vi "Move reports.vi"(11 "source path":path) -> ()   [LabVIEW 2023]
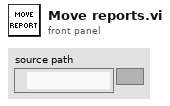
[diagram p1: front panel]
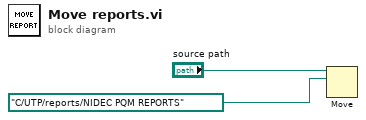
[diagram p0: block diagram]
diagram:
  n1 = Move(source path="source path", 10:path "C:/UTP/reports/NIDEC PQM REPORTS" ("path")) -> ()  [unwired: 3 in, 3 out]
